vi "array smart append -- real.vi"(6 "chunk length":i32=100, 8 "last index":i32, 10 "Numeric":dbl, 11 "Array":dbl[](array[numeric])) -> (0 "last index out":i32, 3 "output array":dbl[](array[numeric]))   [LabVIEW 2021]
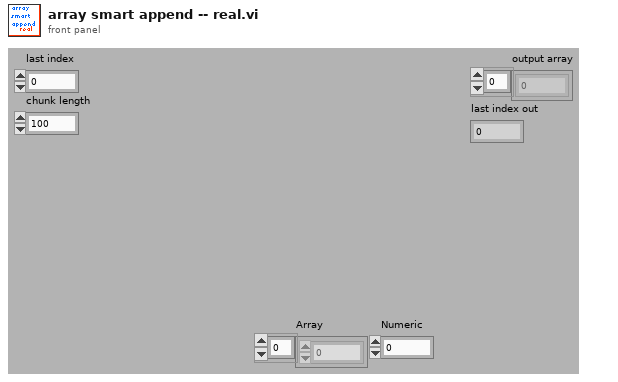
[diagram p1: front panel]
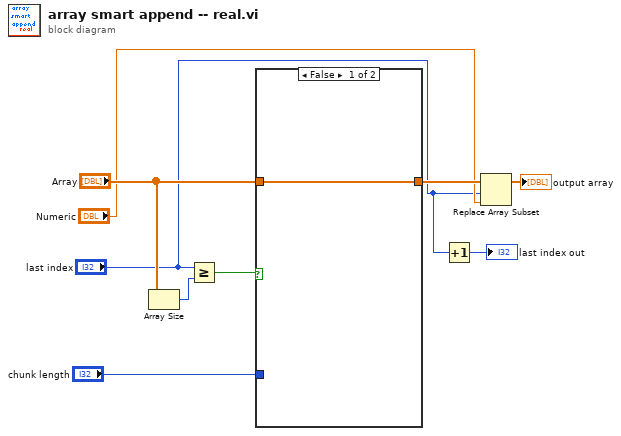
[diagram p0: block diagram]
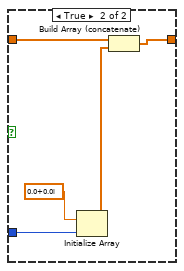
[diagram p2: hidden frame]
diagram:
  n1 = Array Size(array="Array") -> (size(s)=w9:i32)
  n2 = Greater Or Equal?(x="last index", y=w9) -> (x >= y?=w8:bool)
  n3 = case shown="False" w8 {
    tunnel: "Array" -> [w10 w12]
    tunnel: "chunk length" -> [_ w14]
    tunnel: [w10 w11] -> w5
    frame False {
    }
    frame True {
      n4 = Initialize Array(cdb 0.0+0.0i ("element"), w14) -> (w13:cdb[])
      n5 = Build Array (concatenate)(w12, w13) -> (w11:cdb[])
    }
  }
  n6 = Increment(x="last index") -> (x+1=→"last index out":i32)
  n7 = Replace Array Subset(array=w5, new element="Numeric", index="last index") -> (→"output array":cdb[])
